vi "Exp_GetFrameSize.vi"(8 "error in (no error)":errorcluster, 11 "LightField Automation in":refnum<class "LightField Automation.lvclass">) -> (0 "error out":errorcluster, 2 "frame_size":i32[](array[numeric]), 3 "LightField Automation out":refnum<class "LightField Automation.lvclass">)   [LabVIEW 2015, in "LightField Automation.lvclass"]
uses:
  LightField Automation.lvclass
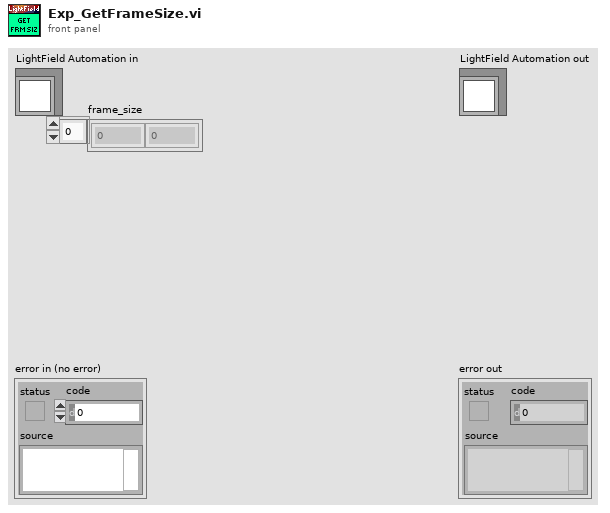
[diagram p1: front panel]
types:
  T1 = cluster{"Image":dbl[][][], "Frame Size":cluster{"F":i32, "Y":i32, "X":i32}}[]
  T2 = cluster{"Image":dbl[][][], "Frame Size":cluster{"F":i32, "Y":i32, "X":i32}}
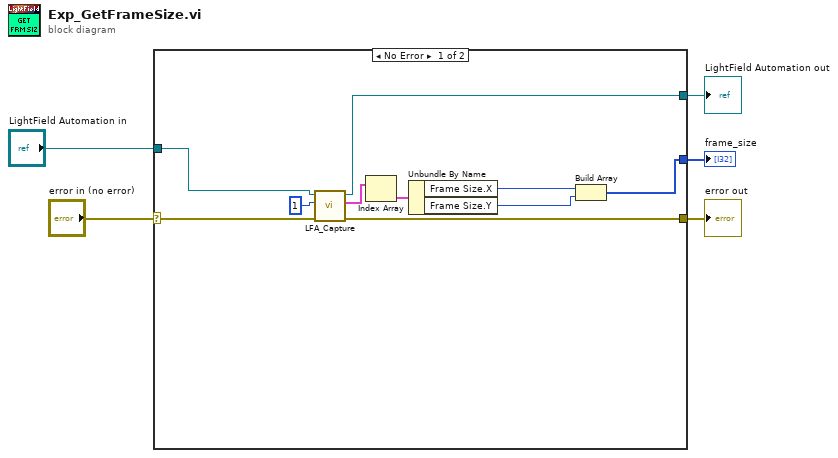
[diagram p0: block diagram]
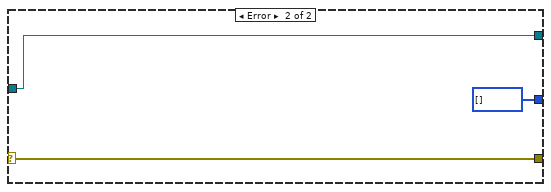
[diagram p2: hidden frame]
diagram:
  n1 = case shown="No Error" "error in (no error)" {
    selector: "error in (no error)" -> [w15 w18]
    tunnel: [w13 w18] -> w4
    tunnel: [w6 w17] -> w2
    tunnel: "LightField Automation in" -> [w12 w17]
    tunnel: [w14 i32[] []] -> w1
    frame No Error {
      n2 = call "LFA_Capture.vi"("error in (no error)"=w15, "Frames"=1, "LightField Automation in"=w12) -> ("error out"=w13:errorcluster, "Data"=w10:T1, "LightField Automation out"=w6:refnum<class "LightField Automation.lvclass">)  [unwired: 6 in]
      n3 = Index Array(array=w10) -> (element=w9:T2)  [unwired: 1 in]
      n4 = Unbundle By Name(w9) -> ("Frame Size.X"=w8:i32, "Frame Size.Y"=w7:i32)
      n5 = Build Array(w8, w7) -> (w14:i32[])
    }
    frame Error {
    }
  }
  "error out" <- w4
  "LightField Automation out" <- w2
  "frame_size" <- w1
